vi "ManualModeNextState.vi"(9 "current state":string="ManualCMD-DirectControl ManualFullOpen>>ManualCMD-MotorStop", 10 "Stop2 Switch":T1={"Tag Name"="S060.PXI.Signals.PlltData.SN", "Network Path"="172.15.51.1,1,0", "use opc"=FALSE, "DataSocket Reference"={"CWDSLib._DCWDataSocket"=refnum, "CWDSLib._DCWData"=refnum, "OnDataUpdated"=0, "OnStatusUpdated"=0}} {"DataSocket Reference"."OnStatusUpdated" format="%.0x"; "DataSocket Reference"."OnDataUpdated" format="%.0x"}, 11 "Stop1 Switch":T1={"Tag Name"="S060.PXI.Signals.PlltData.SN", "Network Path"="172.15.51.1,1,0", "use opc"=FALSE, "DataSocket Reference"={"CWDSLib._DCWDataSocket"=refnum, "CWDSLib._DCWData"=refnum, "OnDataUpdated"=0, "OnStatusUpdated"=0}} {"DataSocket Reference"."OnStatusUpdated" format="%.0x"; "DataSocket Reference"."OnDataUpdated" format="%.0x"}) -> (3 "next state":string)   [LabVIEW 2018]
uses:
  05.UserVI's/type defs/plc path and tag.ctl
  <vilib>/Platform/dataskt.llb/DataSocket Reference Type.ctl
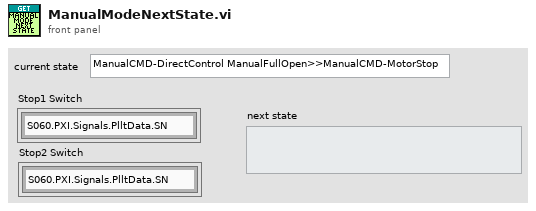
[diagram p1: front panel]
types:
  T1 = typedef "plc path and tag.ctl" = cluster{"Tag Name":string, "Network Path":string, "use opc":bool, "DataSocket Reference":T2}
  T2 = typedef "DataSocket Reference Type.ctl" = cluster{"CWDSLib._DCWDataSocket":refnum<k7>, "CWDSLib._DCWData":refnum<k7>, "OnDataUpdated":u32, "OnStatusUpdated":u32}
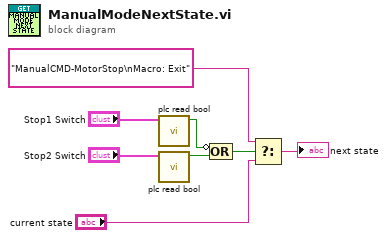
[diagram p0: block diagram]
diagram:
  n1 = call "plc read bool.vi"("addr,tag"="Stop1 Switch") -> ("value"=w7:bool)  [unwired: 9 in, 1 out]
  n2 = call "plc read bool.vi"("addr,tag"="Stop2 Switch") -> ("value"=w8:bool)  [unwired: 9 in, 1 out]
  n3 = Compound Arithmetic op=OR ("复合运算")(invert w7, w8) -> (w6:bool)
  n4 = Select(t="ManualCMD-MotorStop\nMacro: Exit", s=w6, f="current state") -> (s? t:f=→"next state":string)
